vi "DWF FGEN Write DtoA.vi"(3 "Error In":errorcluster caption="Error In (no error)", 4 "Raw Data":i32, 5 "Instrument Handle In":u32) -> (0 "Error Out":errorcluster, 1 "Instrument Handle Out":u32)   [LabVIEW 2024]
doc: "Configures the instrument to output a standard waveform. Any unwired configuration terminals do not change the existing values of those parameters."
uses:
  dwf.dll
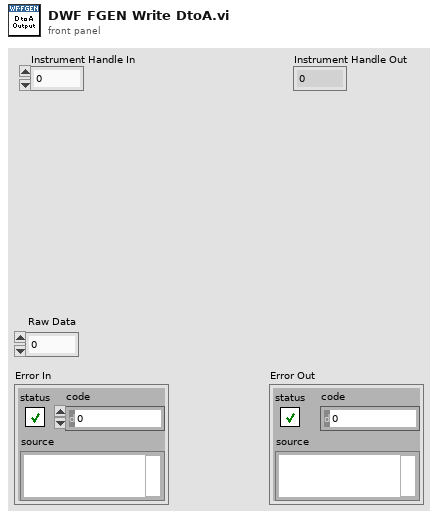
[diagram p1: front panel]
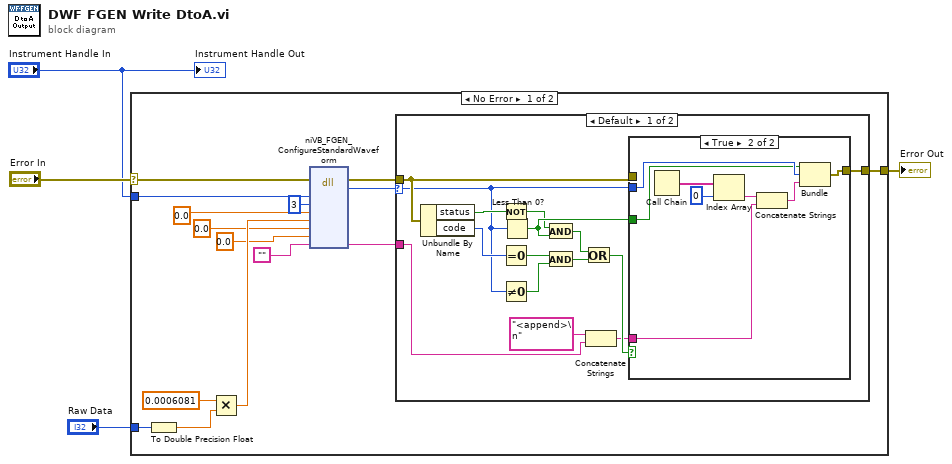
[diagram p0: block diagram]
diagram:
  n1 = case "outter_case" shown="No Error" "Error In" {
    selector: "Error In" -> [w18 w45]
    tunnel: [w19 w45] -> w3
    tunnel: "Instrument Handle In" -> [w15 _]
    tunnel: "Raw Data" -> [w5 _]
    frame No Error {
      n2 = To Double Precision Float(number=w5) -> (double precision float=w6:dbl)
      n3 = Multiply(x=0.0006081, y=w6) -> (x*y=w11:dbl)
      n4 = dll-call lib="dwf.*" fn="niVB_FGEN_ConfigureStandardWaveform"(error in=w18, "instrumentHandle"=w15, "waveformFunction"=u32 3, "amplitude"=0.0, "dcOffset"=w11, "frequency"=0.0, "dutyCycle"=0.0, "szError"="") -> (error out=w17:errorcluster, "return type"=w16:i32, "szError"=w13:string)  [unwired: 8 in, 1 out]
      n5 = case "inner_case" shown="Default" w16 {
        selector: w16 -> [w24 _]
        tunnel: w17 -> [w25 w44]
        tunnel: [w21 w44] -> w19
        tunnel: w13 -> [w20 _]
        frame Default {
          n6 = Unbundle By Name(w25) -> ("status"=w29:bool, "code"=w33:i32)
          n7 = Not(x=w29) -> (.not. x?=w32:bool)
          n8 = Equal To 0?(x=w33) -> (x = 0?=w28:bool)
          n9 = Not Equal To 0?(x=w24) -> (x != 0?=w31:bool)
          n10 = Less Than 0?(x=w24) -> (x < 0?=w34:bool)
          n11 = And(x=w32, y=w34) -> (x .and. y?=w30:bool)
          n12 = And(x=w28, y=w31) -> (x .and. y?=w27:bool)
          n13 = Or(x=w30, y=w27) -> (x .or. y?=w26:bool)
          n14 = Concatenate Strings("<append>\n" ("string"), w20) -> (w23:string)
          n15 = case shown="True" w26 {
            tunnel: [w35 w42] -> w21
            tunnel: w24 -> [_ w41]
            tunnel: w34 -> [_ w40]
            tunnel: w25 -> [w35 _]
            tunnel: w23 -> [_ w36]
            frame False {
            }
            frame True {
              n16 = Call Chain() -> (call chain=w39:string[])
              n17 = Index Array(array=w39, index=0) -> (element=w38:string)
              n18 = Concatenate Strings(w38, w36) -> (w43:string)
              n19 = Bundle(w40, "return type"=w41, w43) -> (w42:cluster{bool, "return type":i32, string})  [unwired: 1 out]
            }
          }
        }
        frame 0 {
        }
      }
    }
    frame Error {
    }
  }
  "Error Out" <- w3
  "Instrument Handle Out" <- "Instrument Handle In"
